vi "Example_circ_buff.vi"() -> ()   [LabVIEW 2021]
panel:
  in  "frames number":i32
  in  "exp_time":u16=100
  out "error out":errorcluster
  out "camera handle":i16
  out "camera name":string
  in  "error in (no error)":errorcluster
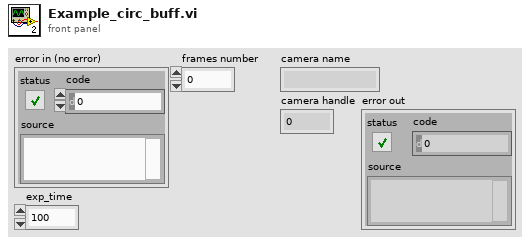
[diagram p1: front panel]
types:
  T1 = enum16{"ATTR_CURRENT", "ATTR_COUNT", "ATTR_TYPE", "ATTR_MIN", "ATTR_MAX", "ATTR_DEFAULT", "ATTR_INCREMENT", "ATTR_ACCESS", "ATTR_AVAIL"}
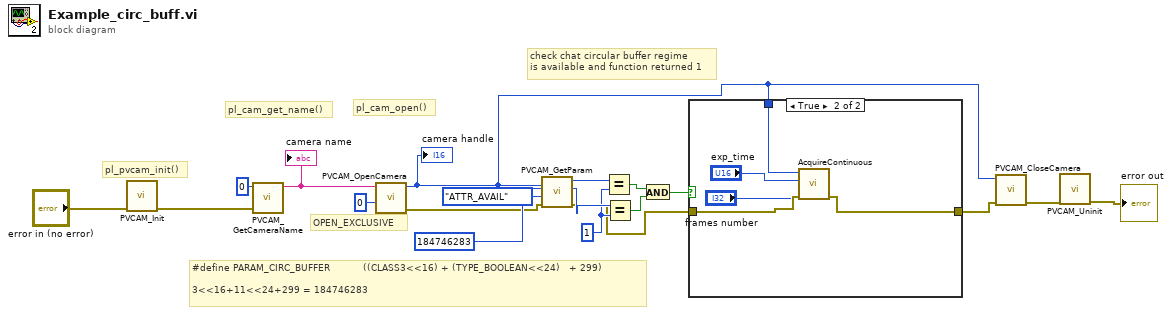
[diagram p0: block diagram]
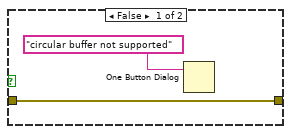
[diagram p2: hidden frame]
diagram:
  w8 = i16 1 ("y")
  # "check chat circular buffer regime \nis available and function returned 1"
  # "#define PARAM_CIRC_BUFFER           ((CLASS3<<16) + (TYPE_BOOLEAN<<24)   + 299)\n\n3<<16+11<<24+299 = 184746283"
  # "OPEN_EXCLUSIVE"
  # "pl_cam_open()"
  # "pl_cam_get_name()"
  # "pl_pvcam_init()"
  n1 = call "PVCAM_Init.vi"("error in (no error)"="error in (no error)") -> ("error out"=w15:errorcluster)  [unwired: 9 in, 1 out]
  n2 = call "PVCAM_GetCameraName.vi"("error in (no error)"=w15, "index in"=i16 0) -> ("string"=w16:string)  [unwired: 6 in, 3 out]
  "camera name" <- w16
  n3 = call "PVCAM_OpenCamera.vi"("mode"=i16 0, "cameraName"=w16) -> ("error out"=w12:errorcluster, "hCam out"=w1:i16)  [unwired: 7 in, 1 out]
  "camera handle" <- w1
  n4 = call "PVCAM_GetParam.vi"("error in (no error)"=w12, "param_attrib"=T1."ATTR_AVAIL", "param_id"=u32 184746283, "hCam"=w1) -> ("error out"=w3:errorcluster, "return type"=w9:i16, "param_value"=w11:i16)  [unwired: 5 in]
  n5 = Equal?(x=w11, y=w8) -> (x = y?=w10:bool)
  n6 = Equal?(x=w9, y=w8) -> (x = y?=w7:bool)
  n7 = And(x=w10, y=w7) -> (x .and. y?=w14:bool)
  n8 = case shown="True" w14 {
    tunnel: w3 -> [w20 w24]
    tunnel: [w20 w23] -> w2
    tunnel: w1 -> [_ w26]
    frame False {
      n9 = One Button Dialog(message="circular buffer not supported") -> ()  [unwired: 1 in, 1 out]
    }
    frame True {
      n10 = call "AcquireContinuous.vi"("error in (no error)"=w24, "frames number"="frames number", "exp_time"="exp_time", "hCam"=w26) -> ("error out"=w23:errorcluster)  [unwired: 6 in, 1 out]
    }
  }
  n11 = call "PVCAM_CloseCamera.vi"("error in (no error)"=w2, "hCam"=w1) -> ("error out"=w6:errorcluster)  [unwired: 8 in, 1 out]
  n12 = call "PVCAM_Uninit.vi"("error in (no error)"=w6) -> ("error out"=→"error out":errorcluster)  [unwired: 9 in, 1 out]
